vi "remove control module.vi"(7 "engine in":refnum<class "engine configuration.lvclass">, 8 "error in":errorcluster, 9 "owner id":string, 10 "name":string, 11 "user module configuration in":refnum<class "user tag bus module configuration.lvclass">) -> (0 "error out":errorcluster, 3 "user module configuration out":refnum<class "user tag bus module configuration.lvclass">, 5 "engine out":refnum<class "engine configuration.lvclass">)   [LabVIEW 2013, in "user tag bus module configuration.lvclass"]
uses:
  user tag bus module configuration.lvclass
  <vilib>/NI/Module Execution Interface/Engine Configuration/engine configuration.lvclass
  user tag bus module configuration.lvclass/user tag bus module configuration.ctl
  <vilib>/NI/Tag Bus Module Framework/root configuration/TBM configuration.lvclass
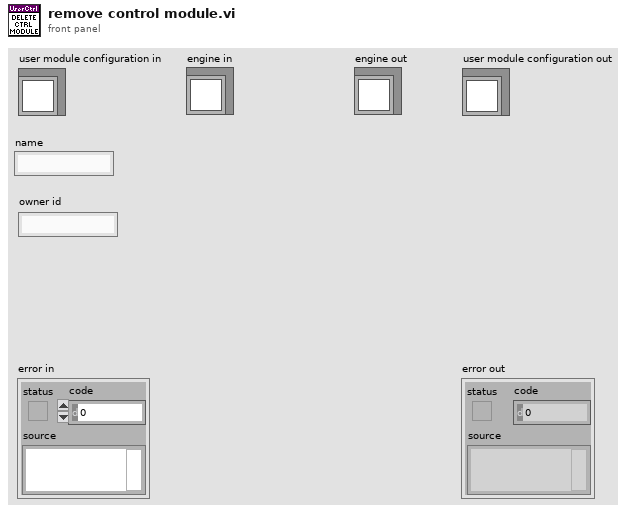
[diagram p1: front panel]
types:
  T1 = typedef "user tag bus module configuration.lvclass/control module configuration.ctl" = cluster{"name":string, "setpoint":refnum<class "TBM channel.lvclass">, "process variable":refnum<class "TBM channel.lvclass">, "output":refnum<class "TBM channel.lvclass">, "gains":T2, "output range":cluster{"output high":dbl, "output low":dbl}}
  T2 = typedef "user tag bus module configuration.lvclass/gains.ctl" = cluster{"Kp":dbl, "Ki":dbl, "Kd":dbl}
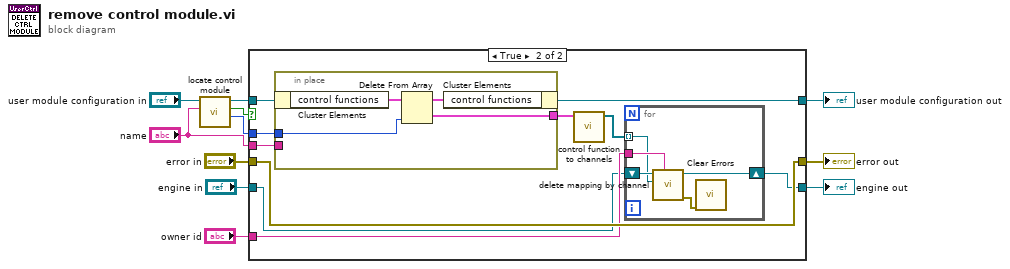
[diagram p0: block diagram]
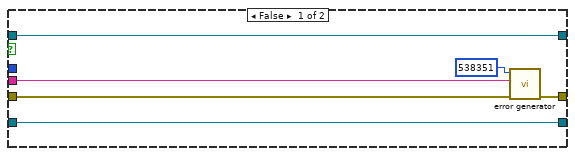
[diagram p2: hidden frame]
diagram:
  n1 = call "locate control module.vi"("name"="name", "user module configuration in"="user module configuration in") -> ("index"=w4:i32, "found"=w9:bool, "user module configuration out"=w10:refnum<class "user tag bus module configuration.lvclass">)  [unwired: 6 in, 1 out]
  n2 = case shown="True" w9 {
    tunnel: w10 -> [w14 w27]
    tunnel: "error in" -> [w17 w23]
    tunnel: [w15 w23] -> w7
    tunnel: [w14 w26] -> w6
    tunnel: "name" -> [w13 w25]
    tunnel: w4 -> [_ w24]
    tunnel: "engine in" -> [w12 w21]
    tunnel: "owner id" -> [_ w22]
    tunnel: [w12 w20] -> w1
    frame False {
      n3 = call <vilib>:"error generator.vi"("error in"=w17, "append error message"=w13, "error code (0)"=538351) -> ("error out"=w15:errorcluster)  [unwired: 8 in]
    }
    frame True {
      n4 = in-place {
        in-place-border: w25 -> [_]
        in-place-border: w24 -> [w34]
        in-place-border: [w33] -> w18
        n5 = in-place-cluster #1(w27) -> ("control functions"=w36:T1[])
        n6 = Delete From Array(array=w36, index=w34) -> (deleted portion=w33:T1, array with subset deleted=w35:T1[])  [unwired: 1 in]
        n7 = in-place-cluster #1("control functions"=w35) -> (w26:refnum<class "user tag bus module configuration.lvclass">)
      }
      n8 = call "control function to channels.vi"("control module configuration"=w18) -> ("channels"=w19:refnum<class "TBM channel.lvclass">[])  [unwired: 10 in]
      n9 = for {
        tunnel: w22 -> [w32]
        shift-right: [w31] -> w20
        shift-left: w21 -> [w29]
        tunnel: w19 -> [w28] mode=indexing
        n10 = call <vilib>:"delete mapping by channel.vi"("owner ID"=w32, "channel"=w28, "engine configuration in"=w29) -> ("error out"=w30:errorcluster, "engine configuration out"=w31:refnum<class "engine configuration.lvclass">)  [unwired: 7 in]
        n11 = call <vilib>:"Clear Errors.vi"("error in (no error)"=w30) -> ()  [unwired: 6 in, 1 out]
      }
    }
  }
  "error out" <- w7
  "user module configuration out" <- w6
  "engine out" <- w1
